vi "ObjectHandler.ExitAll.vi"(8 "error in":errorcluster, 11 "ObjectHandler in":refnum<class "ObjectHandler.lvclass">) -> (0 "error out":errorcluster, 3 "ObjectHandler out":refnum<class "ObjectHandler.lvclass">)   [LabVIEW 2016, in "ObjectHandler.lvclass"]
uses:
  ObjectHandler.lvclass
  ObjectHandler.ObjectWType.ctl
  ObjectHandler.ObjectType.ctl
  ObjectHandler.lvclass/ObjectHandler.ctl
  ViHandler/ViHandler.lvclass
  Package ErrorHandling/ErrorHandling.lvclass
  CentralStorage/CentralStorage.lvclass
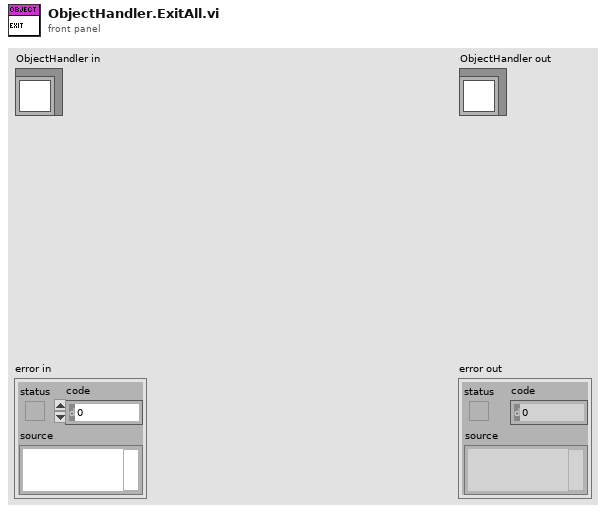
[diagram p1: front panel]
types:
  T1 = typedef "ObjectHandler.lvclass/ObjectHandler.ObjectWType.ctl" = cluster{"ObjectType":T2, "Object":variant}
  T2 = typedef "ObjectHandler.lvclass/ObjectHandler.ObjectType.ctl" = enum16{"undefined", "ObjectHandler", "ViHandler", "ErrorHandler", "CentralStorage", "Hausmodell", "Sondenmodell", "Wärmepumpe", "Umgebung"}
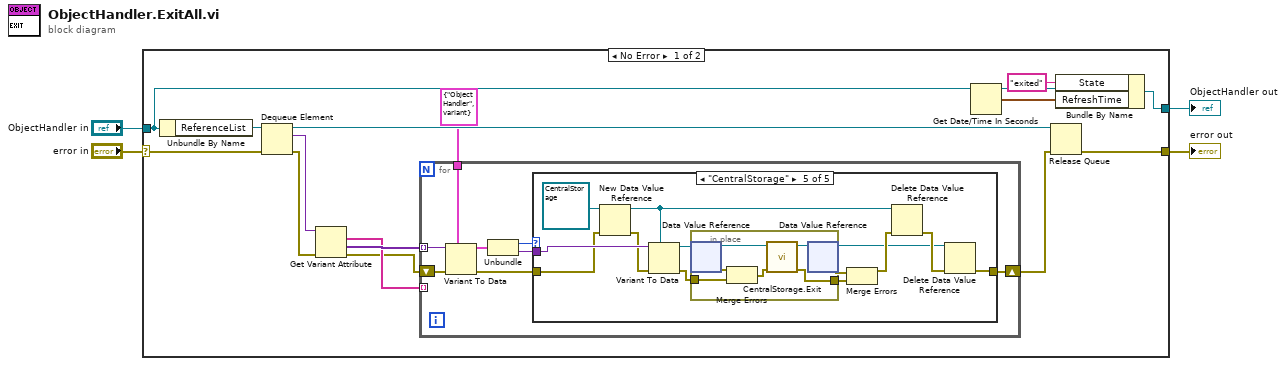
[diagram p0: block diagram]
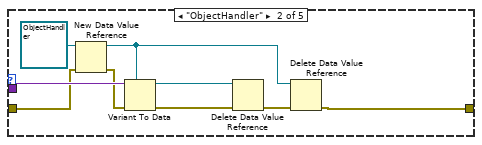
[diagram p3: hidden frame]
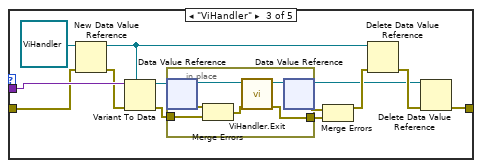
[diagram p4: hidden frame]
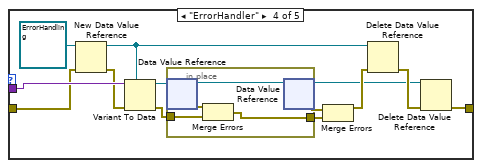
[diagram p5: hidden frame]
diagram:
  n1 = case shown="No Error" "error in" {
    selector: "error in" -> [w17 w94]
    tunnel: [w5 w94] -> w3
    tunnel: [w11 w93] -> w1
    tunnel: "ObjectHandler in" -> [w8 w93]
    frame No Error {
      n2 = Unbundle By Name(w8) -> ("ReferenceList"=w19:refnum<queue>)
      n3 = Dequeue Element(queue=w19, error in (no error)=w17) -> (queue out=w18:refnum<queue>, element=w16:variant, error out=w15:errorcluster)  [unwired: 1 in, 1 out]
      n4 = Get Variant Attribute(Variant=w16, error in=w15) -> (names=w13:string[], values=w14:variant[], error out=w7:errorcluster)  [unwired: 2 in, 1 out]
      n5 = for {
        tunnel: w14 -> [w27] mode=indexing
        tunnel: w13 -> [_] mode=indexing
        tunnel: T1 {"ObjectType"=enum."ObjectHandler", "Object"=variant(refnum<data-value> refnum)} ("ObjectWType") -> [w26]
        shift-right: [w21] -> w6
        shift-left: w7 -> [w24]
        n6 = Variant To Data(error in=w24, type=w26, Variant=w27) -> (data=w25:T1, error out=w20:errorcluster)
        n7 = Unbundle(w25) -> ("ObjectType"=w22:T2, "Object"=w23:variant)
        n8 = case shown="\"CentralStorage\"" w22 {
          tunnel: w23 -> [_ w36 w50 w69 w86]
          tunnel: w20 -> [w28 w34 w48 w67 w84]
          tunnel: [w28 w29 w45 w64 w81] -> w21
          frame "undefined", Default {
          }
          frame "ObjectHandler" {
            n9 = New Data Value Reference(data value=refnum<class "ObjectHandler.lvclass"> refnum ("ObjectHandler.lvclass"), error in=w34) -> (data value reference=w33:refnum<data-value>, error out=w35:errorcluster)
            n10 = Variant To Data(error in=w35, type=w33, Variant=w36) -> (data=w32:refnum<data-value>, error out=w31:errorcluster)
            n11 = Delete Data Value Reference(data value reference=w32, error in=w31) -> (error out=w30:errorcluster)  [unwired: 1 out]
            n12 = Delete Data Value Reference(data value reference=w33, error in=w30) -> (error out=w29:errorcluster)  [unwired: 1 out]
          }
          frame "ViHandler" {
            n13 = New Data Value Reference(data value=refnum<class "ViHandler.lvclass"> refnum ("ViHandler.lvclass"), error in=w48) -> (data value reference=w47:refnum<data-value>, error out=w49:errorcluster)
            n14 = Variant To Data(error in=w49, type=w47, Variant=w50) -> (data=w44:refnum<data-value>, error out=w43:errorcluster)
            n15 = in-place {
              in-place-border: w43 -> [w55]
              in-place-border: [w51] -> w41
              n16 = in-place-dvr #1(w44) -> (w54:refnum<class "ViHandler.lvclass">, w56:errorcluster)
              n17 = Merge Errors(w56, w55) -> (w52:errorcluster)
              n18 = call "ViHandler.Exit.vi"("error in (no error)"=w52, "ViHandler in"=w54) -> ("error out"=w51:errorcluster, "ViHandler out"=w53:refnum<class "ViHandler.lvclass">)  [unwired: 8 in]
              n19 = in-place-dvr #1(w53) -> (w38:refnum<data-value>, w42:errorcluster)
            }
            n20 = Merge Errors(w42, w41) -> (w40:errorcluster)
            n21 = Delete Data Value Reference(data value reference=w47, error in=w40) -> (error out=w46:errorcluster)  [unwired: 1 out]
            n22 = Delete Data Value Reference(data value reference=w38, error in=w46) -> (error out=w45:errorcluster)  [unwired: 1 out]
          }
          frame "ErrorHandler" {
            n23 = New Data Value Reference(data value=refnum<class "ErrorHandling.lvclass"> refnum ("ErrorHandling.lvclass"), error in=w67) -> (data value reference=w66:refnum<data-value>, error out=w68:errorcluster)
            n24 = Variant To Data(error in=w68, type=w66, Variant=w69) -> (data=w63:refnum<data-value>, error out=w62:errorcluster)
            n25 = in-place {
              in-place-border: w62 -> [w72]
              in-place-border: [w70] -> w60
              n26 = in-place-dvr #2(w63) -> (w71:refnum<class "ErrorHandling.lvclass">, w73:errorcluster)
              n27 = Merge Errors(w73, w72) -> (w70:errorcluster)
              n28 = in-place-dvr #2(w71) -> (w58:refnum<data-value>, w61:errorcluster)
            }
            n29 = Merge Errors(w61, w60) -> (w59:errorcluster)
            n30 = Delete Data Value Reference(data value reference=w66, error in=w59) -> (error out=w65:errorcluster)  [unwired: 1 out]
            n31 = Delete Data Value Reference(data value reference=w58, error in=w65) -> (error out=w64:errorcluster)  [unwired: 1 out]
          }
          frame "CentralStorage" {
            n32 = New Data Value Reference(data value=refnum<class "CentralStorage.lvclass"> refnum ("CentralStorage.lvclass"), error in=w84) -> (data value reference=w83:refnum<data-value>, error out=w85:errorcluster)
            n33 = Variant To Data(error in=w85, type=w83, Variant=w86) -> (data=w80:refnum<data-value>, error out=w79:errorcluster)
            n34 = in-place {
              in-place-border: w79 -> [w91]
              in-place-border: [w88] -> w77
              n35 = in-place-dvr #3(w80) -> (w90:refnum<class "CentralStorage.lvclass">, w92:errorcluster)
              n36 = Merge Errors(w92, w91) -> (w87:errorcluster)
              n37 = call "CentralStorage.Exit.vi"("error in (no error)"=w87, "CentralStorage in"=w90) -> ("error out"=w88:errorcluster, "CentralStorage out"=w89:refnum<class "CentralStorage.lvclass">)  [unwired: 8 in]
              n38 = in-place-dvr #3(w89) -> (w75:refnum<data-value>, w78:errorcluster)
            }
            n39 = Merge Errors(w78, w77) -> (w76:errorcluster)
            n40 = Delete Data Value Reference(data value reference=w83, error in=w76) -> (error out=w82:errorcluster)  [unwired: 1 out]
            n41 = Delete Data Value Reference(data value reference=w75, error in=w82) -> (error out=w81:errorcluster)  [unwired: 1 out]
          }
        }
      }
      n42 = Get Date/Time In Seconds() -> (seconds since 1Jan1904=w9:timestamp)
      n43 = Release Queue(queue=w18, error in (no error)=w6) -> (error out=w5:errorcluster)  [unwired: 1 in, 2 out]
      n44 = Bundle By Name(cluster=w8, "State"="exited", "RefreshTime"=w9) -> (w11:refnum<class "ObjectHandler.lvclass">)
    }
    frame Error {
    }
  }
  "error out" <- w3
  "ObjectHandler out" <- w1
